vi "Get Server Internal UEs.vi"(11 "OOP Server in":refnum<class "OCVServer.lvclass">) -> (2 "Server Internal UEs":T1, 3 "OOP Server out":refnum<class "OCVServer.lvclass">)   [LabVIEW 2019, in "OCVServer.lvlib" / "OCVServer.lvclass"]
uses:
  OCVServer.lvclass
  typeDefs/Server Internal UEs.ctl
  typeDefs/Server Internal Message UE.ctl
  typeDefs/Server Internal Message.ctl
  OCVServer.lvclass/OCVServer.ctl
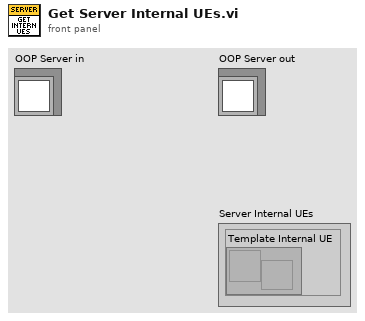
[diagram p1: front panel]
types:
  T1 = typedef "OCVServer.lvlib/OCVServer.lvclass/Server Internal UEs.ctl" = cluster{"Template Internal UE":T2}
  T2 = typedef "OCVServer.lvlib/OCVServer.lvclass/Server Internal Message UE.ctl" = refnum<user-event>
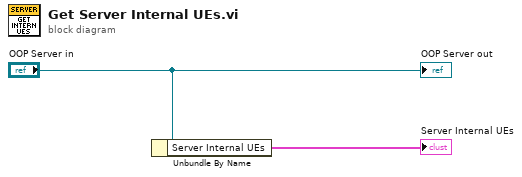
[diagram p0: block diagram]
diagram:
  n1 = Unbundle By Name("OOP Server in") -> ("Server Internal UEs"=→"Server Internal UEs":T1)
  "OOP Server out" <- "OOP Server in"
